vi "Set 0 Volts.vi"(7 "Delay_After_Powerdown":dbl format="%#_6p", 8 "error in (no error)":errorcluster, 10 "Pins":string[](array[string])=["VDD", "RF_Bias"], 11 "Semiconductor Module Context":T1) -> (0 "error out":errorcluster)   [LabVIEW 2013]
uses:
  <vilib>/NI_TestStand_SemiconductorModule/NI_TestStand_Semiconductor_Module.lvlibp/PinMap/General/SemiconductorModuleContext.ctl
  <vilib>/NI_TestStand_SemiconductorModule/NI_TestStand_Semiconductor_Module.lvlibp/PinMap/DC Power/PinsToNIDCPowerSessions.vi
  <vilib>/NI_TestStand_SemiconductorModule/NI_TestStand_Semiconductor_Module.lvlibp
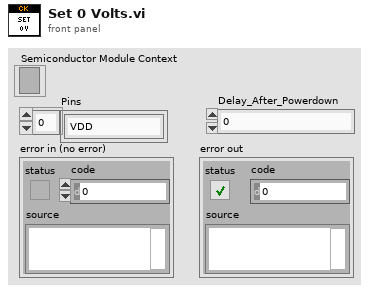
[diagram p1: front panel]
types:
  T1 = typedef "NI_TestStand_Semiconductor_Module.lvlibp/SemiconductorModuleContext.ctl" = refnum<k7>
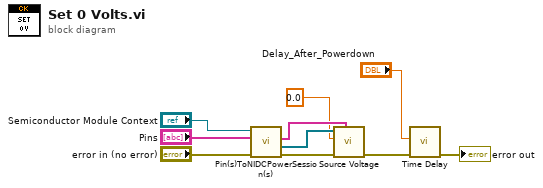
[diagram p0: block diagram]
diagram:
  n1 = call-poly <vilib>:"Pin(s)ToNIDCPowerSession(s).vi"("error in (no error)"="error in (no error)", "Pins"="Pins", "Semiconductor Module Context"="Semiconductor Module Context") -> ("error out"=w8:errorcluster, "Instrument Sessions"=w9:refnum<k15>[], "Channel Lists"=w6:string[])  [unwired: 4 in, 2 out]
  n2 = call "Source Voltage.vi"("Channel Lists"=w6, "error in (no error)"=w8, "voltage level"=0.0, "Instrument Sessions In"=w9) -> ("error out"=w3:errorcluster)  [unwired: 4 in, 3 out]
  n3 = call "Time Delay"("error in (no error)"=w3, "Delay Time (s)"="Delay_After_Powerdown") -> ("error out"=→"error out":errorcluster)  [unwired: 9 in]
